vi "Actualizar Saldo.vi"(8 "error in (no error)":errorcluster, 9 "Saldo":string, 10 "Monedas":T1) -> (0 "error out":errorcluster)   [LabVIEW 2019]
doc: "Dependiendo de las monedas que se agregen el saldo va a estar siendo actualizado\n_____\nCreated using Delacor QMH Event Scripter 5.0.0.112."
uses:
  Actualizar Saldo Argument--cluster.ctl
  Monedas.lvlib
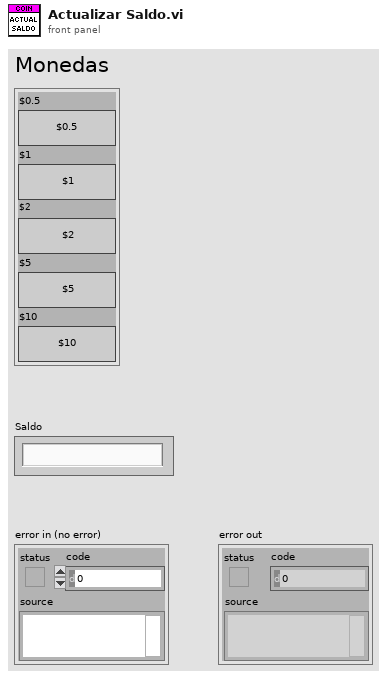
[diagram p1: front panel]
types:
  T1 = cluster{"$0.5":bool, "$1":bool, "$2":bool, "$5":bool, "$10":bool}
  T2 = typedef "Actualizar Saldo Argument--cluster.ctl" = cluster{"Monedas":cluster{"$0.5":bool, "$1":bool, "$2":bool, "$5":bool, "$10":bool}, "Saldo":string}
  T3 = typedef "Monedas.lvlib/Request Events--cluster.ctl" = cluster{"Stop Module":refnum<user-event>, "Show Panel":refnum<user-event>, "Hide Panel":refnum<user-event>, "Get Module Execution Status":refnum<user-event>, "Show Diagram":refnum<user-event>}
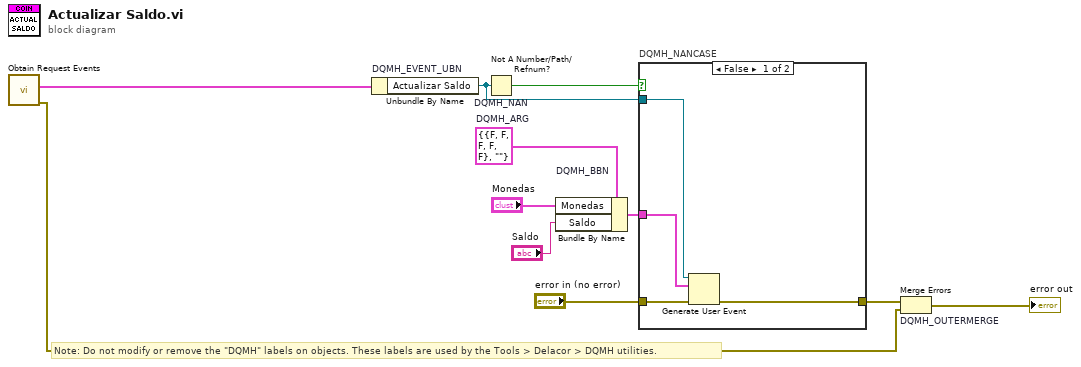
[diagram p0: block diagram]
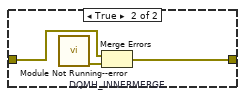
[diagram p2: hidden frame]
diagram:
  w5 = T2 {"Monedas"={"$0.5"=FALSE, "$1"=FALSE, "$2"=FALSE, "$5"=FALSE, "$10"=FALSE}, "Saldo"=""}  # DQMH_ARG
  # "Note: Do not modify or remove the \"DQMH\" labels on objects. These labels are used by the Tools > Delacor > DQMH utilities."
  n1 = call "Obtain Request Events.vi"() -> ("error out"=w2:errorcluster, "Monedas Request Events"=w1:T3)  [unwired: 10 in]
  n2 = Unbundle By Name "DQMH_EVENT_UBN"(w1) -> ("Actualizar Saldo"=w7:refnum<user-event>)
  n3 = Not A Number/Path/Refnum? "DQMH_NAN"(number/path/refnum=w7) -> (NaN/Path/Refnum?=w8:bool)
  n4 = Bundle By Name "DQMH_BBN"(cluster=w5, "Monedas"="Monedas", "Saldo"="Saldo") -> (w9:T2)
  n5 = case "DQMH_NANCASE" shown="False" w8 {
    tunnel: "error in (no error)" -> [w15 w18]
    tunnel: [w14 w17] -> w6
    tunnel: w7 -> [w13 _]
    tunnel: w9 -> [w12 _]
    frame False {
      n6 = Generate User Event(user event=w13, event data cluster=w12, error in=w15) -> (error out=w14:errorcluster)  [unwired: 1 in, 1 out]
    }
    frame True {
      n7 = call "Module Not Running--error.vi"() -> ("error out"=w16:errorcluster)  [unwired: 11 in]
      n8 = Merge Errors "DQMH_INNERMERGE"(w18, w16) -> (w17:errorcluster)
    }
  }
  n9 = Merge Errors "DQMH_OUTERMERGE"(w6, w2) -> (→"error out":errorcluster)
